vi "ReaderReadFrameCore.vi"(7 "Reader Frame Action":T2, 8 "error in (no error)":errorcluster, 9 "Position":dbl, 10 "Greyscale Image":T1, 11 "Handle":refnum<data-value>) -> (0 "error out":errorcluster)   [LabVIEW 2020, in "video_io.lvlib"]
uses:
  video_io.lvlib
  Reader Frame Action.ctl
  image/Greyscale Image.ctl
  common/common.lvlib
  common/bin/gartoolkit_32-1.dll
  image/image.lvlib
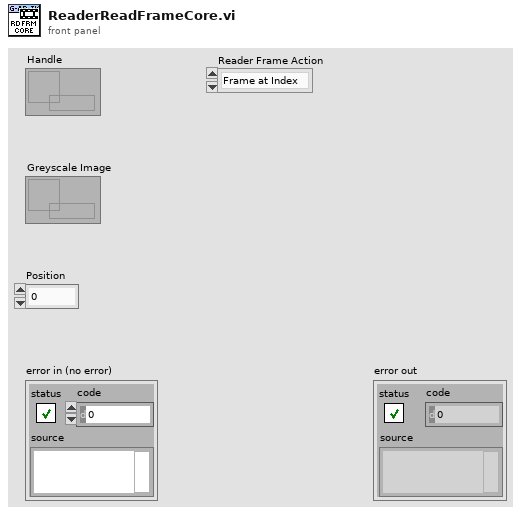
[diagram p1: front panel]
types:
  T1 = typedef "image.lvlib/Greyscale Image.ctl" = refnum<data-value>
  T2 = typedef "video_io.lvlib/Reader Frame Action.ctl" = enum8{"Frame at Index", "Frame at ms", "Next"}
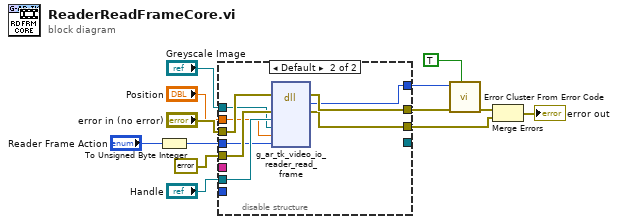
[diagram p0: block diagram]
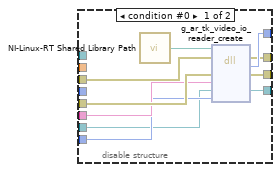
[diagram p2: hidden frame]
diagram:
  n1 = To Unsigned Byte Integer(number="Reader Frame Action") -> (unsigned 8bit integer=w4:u8)
  n2 = disable-structure shown="Default" {
    disable-tunnel: "error in (no error)" -> [w23 w32]
    disable-tunnel: errorcluster {"status"=FALSE, "code"=0, "source"=""} ("error constant") -> [w22 w31]
    disable-tunnel: _ -> [w21 _]
    disable-tunnel: "Handle" -> [w19 w30]
    disable-tunnel: [w15 w29] -> w10
    disable-tunnel: [w17 w28] -> w9
    disable-tunnel: [w16 _] -> _
    disable-tunnel: [w14 w27] -> w7
    disable-tunnel: _ -> [w20 _]
    disable-tunnel: w4 -> [_ w26]
    disable-tunnel: "Position" -> [_ w25]
    disable-tunnel: "Greyscale Image" -> [_ w24]
    frame condition #0 {
      n3 = call "NI-Linux-RT Shared Library Path.vi"() -> ("Path"=w18:path)
      n4 = dll-call lib="?" fn="g_ar_tk_video_io_reader_create" ("g_ar_toolkit.*.*:g_ar_tk_capture_context_create")(path in=w18, error in=w23, "error_cluster"=w22, "Path"=w21, "Handle"=w19, "n_channels"=w20) -> (error out=w15:errorcluster, "return type"=w17:i32, "error_cluster"=w14:errorcluster, "Handle"=w16:refnum<data-value>)  [unwired: 3 in, 1 out]
    }
    frame condition #1 (active) {
      n5 = dll-call lib="C:/serenial/lib/g-augmented-reality-toolkit/LabVIEW/common/bin/gartoolkit_*-1.*" fn="g_ar_tk_video_io_reader_read_frame" ("g_ar_toolkit.*.*:g_ar_tk_capture_context_create")(error in=w32, "error_cluster"=w31, "Handle"=w30, "Image"=w24, "Position"=w25, "Action"=w26) -> (error out=w29:errorcluster, "return type"=w28:i32, "error_cluster"=w27:errorcluster)  [unwired: 6 in, 1 out]
    }
  }
  n6 = call <vilib>:"Error Cluster From Error Code.vi"("show call chain? (False)"=TRUE, "error in (no error)"=w10, "error code (0)"=w9) -> ("error out"=w13:errorcluster)  [unwired: 6 in]
  n7 = Merge Errors(w13, w7) -> (→"error out":errorcluster)
